vi "1.2-Where.vi"   [LabVIEW 2010]
uses:
  2-Low Neurons/2.2-Where Sensor Typedef.ctl
  <vilib>/eio/EIOMethodNode/EIOMethodNode.xnode
  <vilib>/rvi/eio/nirviEIOMethodImplementation/nirviEIOMethodImplementation.xnode
  <vilib>/rvi/eio/common/nirviEmuClasses.ctl
  1.0-Hindbrain Global.vi
  <vilib>/rvi/eio/common/nirviEmuTemplateMethod_noerrors.vi
types:
  T1 = typedef "2.2-Where Sensor Typedef.ctl" = cluster{"INS X":i16, "INS Y":i16, "INS Z":i16, "INS Yaw":i16, "INS Raw":i8}
  T2 = typedef "nirviEmuClasses.ctl" = enum16{"IO Read", "IO Write", "Method", "Property Read", "Property Write"}
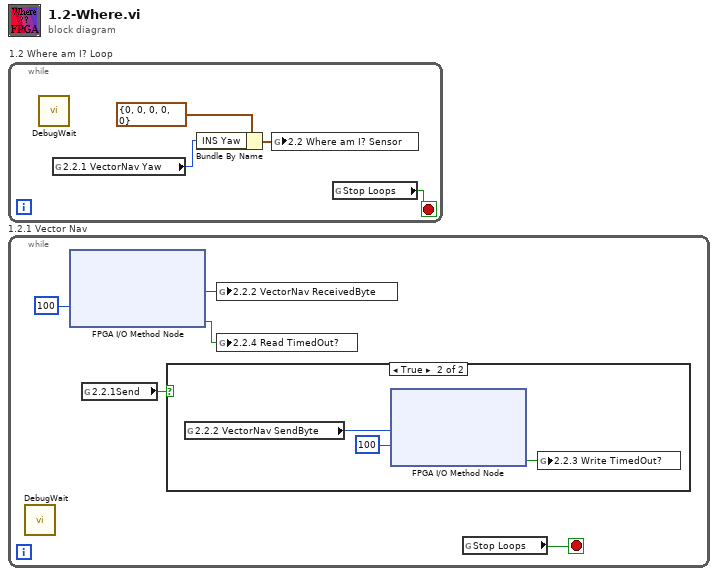
[diagram p0: block diagram]
diagram:
  n1 = while "1.2 Where am I? Loop" {
    stop <- w4 stop-if-true
    n2 = call "DebugWait.vi"() -> ()  [unwired: 12 in]
    n3 = global read "1.0-Hindbrain Global.vi" "2.2.1 VectorNav Yaw"() -> (w2:i16)
    n4 = Bundle By Name(cluster=T1 {"INS X"=0, "INS Y"=0, "INS Z"=0, "INS Yaw"=0, "INS Raw"=0} ("2.2 Where am I? Sensor"), "INS Yaw"=w2) -> (w1:T1)
    n5 = global write "1.0-Hindbrain Global.vi" "2.2 Where am I? Sensor"(w1) -> ()
    n6 = global read "1.0-Hindbrain Global.vi" "Stop Loops"() -> (w4:bool)
  }
  n7 = while "1.2.1 Vector Nav" {
    stop <- w9 stop-if-true
    n8 = call "DebugWait.vi"() -> ()  [unwired: 12 in]
    n9 = xnode "FPGA I/O Method Node"("Timeout (ms)"=100) -> ("Data"=w8:u8, "Timed Out"=w6:bool)  [unwired: 1 in, 1 out]
    n10 = global read "1.0-Hindbrain Global.vi" "2.2.1Send"() -> (w5:bool)
    n11 = case shown="True" w5 {
      frame False {
      }
      frame True {
        n12 = global read "1.0-Hindbrain Global.vi" "2.2.2 VectorNav SendByte"() -> (w11:u8)
        n13 = xnode "FPGA I/O Method Node"("Data"=w11, "Timeout (ms)"=100) -> ("Timed Out"=w10:bool)  [unwired: 1 in, 1 out]
        n14 = global write "1.0-Hindbrain Global.vi" "2.2.3 Write TimedOut?"(w10) -> ()
      }
    }
    n15 = global write "1.0-Hindbrain Global.vi" "2.2.2 VectorNav ReceivedByte"(w8) -> ()
    n16 = global write "1.0-Hindbrain Global.vi" "2.2.4 Read TimedOut?"(w6) -> ()
    n17 = global read "1.0-Hindbrain Global.vi" "Stop Loops"() -> (w9:bool)
  }
